vi "Array to String.vi"(0 "array":string[](array[string]), 1 "delimiter (;)":string=";") -> (2 "string":string)   [LabVIEW 2017]
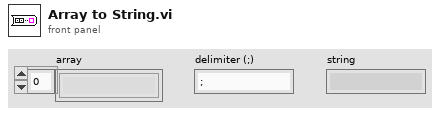
[diagram p1: front panel]
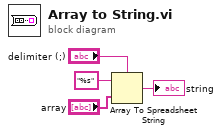
[diagram p0: block diagram]
diagram:
  n1 = Array To Spreadsheet String(delimiter (Tab)="delimiter (;)", array="array", 3:"%s" ("format string")) -> (spreadsheet string=→"string":string)
